vi "test.vi"() -> ()   [LabVIEW 2009]
uses:
  <vilib>/userDefined/High Color/IMAQdx.ctl
  IMAQdx Cam/IMAQdx Cam.lvclass
panel:
  in  "open settings":bool
  in  "stop":bool
  out "Image":T1(plugin-control)
  in  "Camera Name":T2="SRingPumpCamera"
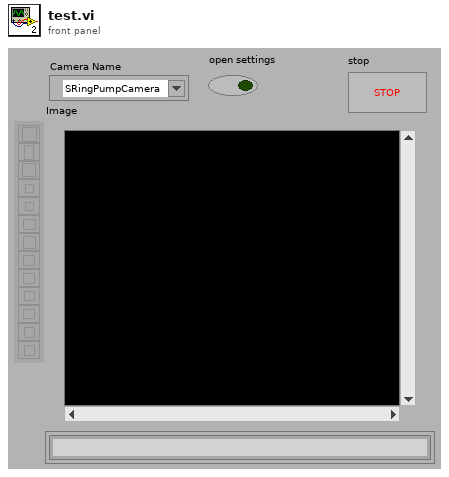
[diagram p1: front panel]
types:
  T1 = typedef "IMAQ Image.ctl" = refnum<image>
  T2 = typedef "IMAQdx.ctl" = refnum<k21>
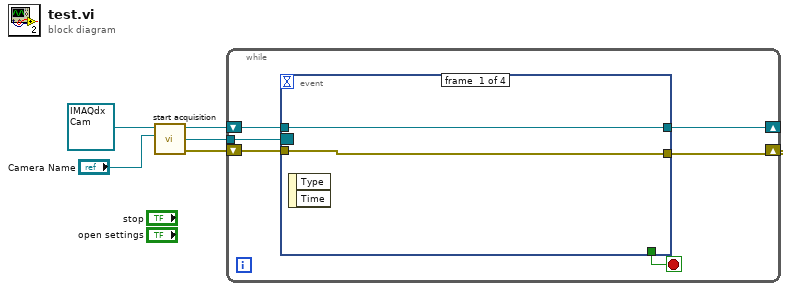
[diagram p0: block diagram]
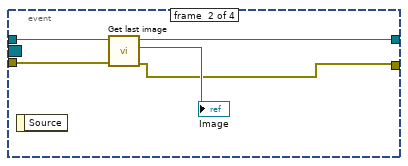
[diagram p2: hidden frame]
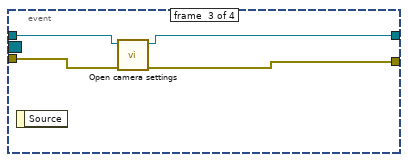
[diagram p3: hidden frame]
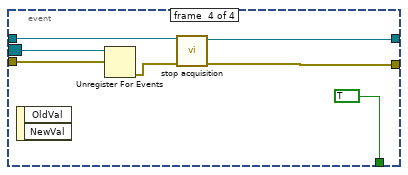
[diagram p4: hidden frame]
diagram:
  n1 = call-dynamic "start acquisition.vi"("Camera Name"="Camera Name", "IMAQdx Cam in"=refnum<class "IMAQdx Cam.lvclass"> refnum ("IMAQdx Cam.lvclass")) -> ("error out"=w2:errorcluster, "Event Registration Refnum"=w1:refnum<event-registration>, "IMAQdx Cam out"=w3:refnum<class "IMAQdx Cam.lvclass">)  [unwired: 7 in]
  n2 = while {
    tunnel: w1 -> [w6]
    shift-right: [w9] -> _
    shift-left: w3 -> [w11]
    shift-right: [w8] -> _
    shift-left: w2 -> [w10]
    stop <- w7 stop-if-true
    n3 = event shown="[1] <Session Out>: FrameDone" {
      selector: w6 -> [_ _ _ w28]
      dyn-events: _ -> [_ _ _ _]
      timeout: _ -> [_ _ _ _]
      tunnel: w11 -> [w12 w18 w22 w26]
      tunnel: w10 -> [w13 w17 w21 w27]
      tunnel: [w12 w15 w19 w24] -> w9
      tunnel: [w13 w14 w20 w23] -> w8
      tunnel: [_ _ _ TRUE] -> w7
      event #0 {
        n4 = event-data() -> ()  [unwired: 1 in, 2 out]
      }
      event #1 {
        n5 = event-data() -> ()  [unwired: 1 in, 1 out]
        n6 = call-dynamic "Get last image.vi"("error in (no error)"=w17, "IMAQdx Cam in"=w18) -> ("error out"=w14:errorcluster, "Image Out"=→"Image":T1, "IMAQdx Cam out"=w15:refnum<class "IMAQdx Cam.lvclass">)  [unwired: 7 in]
      }
      event #2 {
        n7 = event-data() -> ()  [unwired: 1 in, 1 out]
        n8 = call-dynamic "Open camera settings.vi"("error in (no error)"=w21, "IMAQdx Cam in"=w22) -> ("error out"=w20:errorcluster, "IMAQdx Cam out"=w19:refnum<class "IMAQdx Cam.lvclass">)  [unwired: 8 in]
      }
      event #3 {
        n9 = event-data() -> ()  [unwired: 1 in, 2 out]
        n10 = Unregister For Events(event registration refnum=w28, error in=w27) -> (error out=w25:errorcluster)
        n11 = call-dynamic "stop acquisition.vi"("error in (no error)"=w25, "IMAQdx Cam in"=w26) -> ("error out"=w23:errorcluster, "IMAQdx Cam out"=w24:refnum<class "IMAQdx Cam.lvclass">)  [unwired: 8 in]
      }
    }
  }
